vi "Find Tag From Channel Name.vi"(10 "channel name":string, 11 "Module Mappings":T1) -> (2 "found?":bool, 3 "mapped tag":string)   [LabVIEW 2013, in "Engine Runtime Interface.lvclass"]
uses:
  Engine Runtime Interface.lvclass
  Engine Configuration/Module Mappings.ctl
  <vilib>/NI/Tag Bus/table/mapping specification.ctl
  <vilib>/NI/Tag Bus/tag/Data Type.ctl
  <vilib>/NI/Tag Bus/table/mapping.ctl
  <vilib>/NI/Tag Bus/tag/tag descriptor.lvclass
  Engine Configuration/engine configuration.lvclass
  <vilib>/NI/Tag Bus/table/data table.lvlib
panel:
  out "instance name":string
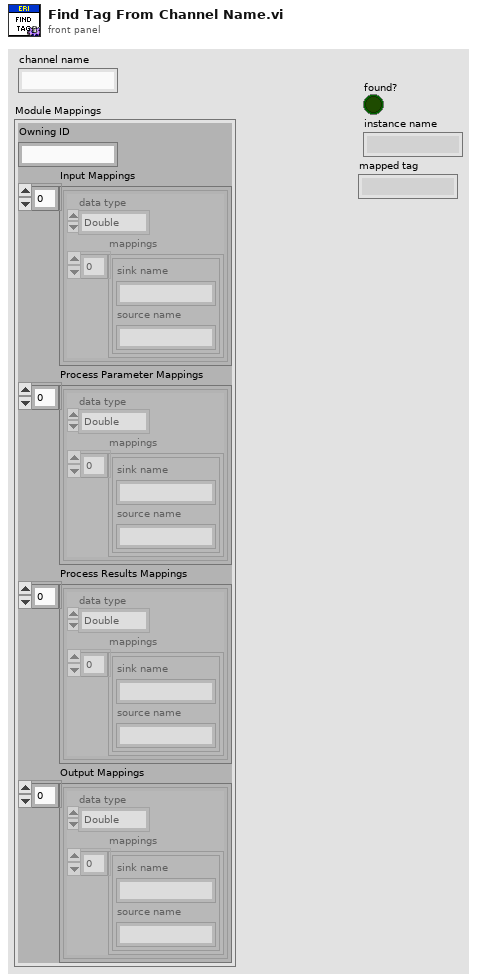
[diagram p1: front panel]
types:
  T1 = typedef "engine configuration.lvclass/Module Mappings.ctl" = cluster{"Owning ID":string, "Input Mappings":T2[], "Process Parameter Mappings":T2[], "Process Results Mappings":T2[], "Output Mappings":T2[]}
  T2 = typedef "tag bus.lvlib/data table.lvlib/mapping specification.ctl" = cluster{"data type":T3, "mappings":T4[]}
  T3 = typedef "tag bus.lvlib/tag descriptor.lvclass/Data Type.ctl" = enum16{"Double", "Single", "I64", "I32", "I16", "I8", "U64", "U32", "U16", "U8", "Boolean", "String", "Array of Double", "Array of Single", "Array of I64", "Array of I32", "Array of I16", "Array of I8", "Array of U64", "Array of U32", "Array of U16", "Array of U8", "Array of Boolean", "Array of String"}
  T4 = typedef "tag bus.lvlib/data table.lvlib/mapping.ctl" = cluster{"sink name":string, "source name":string}
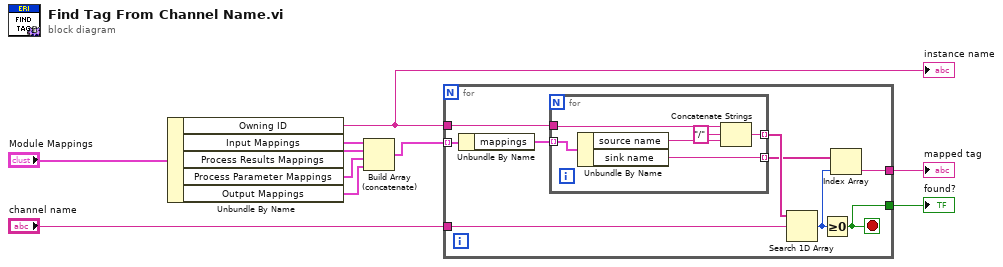
[diagram p0: block diagram]
diagram:
  n1 = Unbundle By Name("Module Mappings") -> ("Owning ID"=w10:string, "Input Mappings"=w8:T2[], "Process Results Mappings"=w7:T2[], "Process Parameter Mappings"=w6:T2[], "Output Mappings"=w5:T2[])
  "instance name" <- w10
  n2 = Build Array (concatenate)(w8, w7, w6, w5) -> (w4:T2[])
  n3 = for {
    tunnel: w4 -> [w19] mode=indexing
    tunnel: w10 -> [w17]
    tunnel: "channel name" -> [w15]
    tunnel: [w13] -> w1
    tunnel: [w12] -> w3
    stop <- w12 stop-if-true
    n4 = Unbundle By Name(w19) -> ("mappings"=w18:T4[])
    n5 = for {
      tunnel: w18 -> [w25] mode=indexing
      tunnel: w17 -> [w23]
      tunnel: [w21] -> w16 mode=indexing
      tunnel: [w20] -> w11 mode=indexing
      n6 = Unbundle By Name(w25) -> ("source name"=w22:string, "sink name"=w20:string)
      n7 = Concatenate Strings(w23, "/" ("string"), w22) -> (w21:string)
    }
    n8 = Search 1D Array(1D array=w16, element=w15) -> (index of element=w14:i32)  [unwired: 1 in]
    n9 = Greater Or Equal To 0?(x=w14) -> (x >= 0?=w12:bool)
    n10 = Index Array(array=w11, index=w14) -> (element=w13:string)
  }
  "found?" <- w3
  "mapped tag" <- w1
